vi "test Total Channel Count.vi"(8 "error in (no error)":errorcluster, 11 "TestCase in":refnum<class "Configuration Tests.lvclass">) -> (0 "error out":errorcluster, 3 "TestCase out":refnum<class "Configuration Tests.lvclass">)   [LabVIEW 2017, in "Configuration Tests.lvclass"]
uses:
  Configuration Tests.lvclass
  Mock Classes/Transfer/Mock Transfer.lvclass
  C:/github/data-sharing-framework/Data Sharing Framework Core/Engine/Classes/Transfer/Transfer.lvclass
  Configuration/Public/Controls/DSF Engine Channel Configuration.ctl
  Configuration/Public/Controls/DSF Data Type.ctl
  <vilib>/addons/_JKI Toolkits/VI Tester/TestCase.llb/TestCase.lvclass
  Engine/Classes/Transfer/Transfer.lvclass
  DSF Core.lvlib
  C:/Program Files (x86)/National Instruments/LabVIEW 2017/vi.lib/addons/_JKI Toolkits/VI Tester/TestCase.llb/TestCase.lvclass
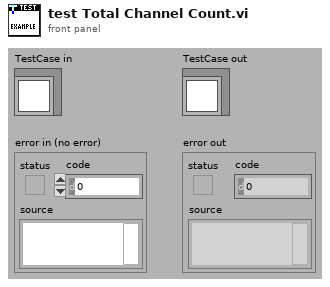
[diagram p1: front panel]
types:
  T1 = typedef "DSF Core.lvlib/DSF Engine Channel Configuration.ctl" = cluster{"engine offset":u64, "name":string, "data type":T2, "count":u64, "buffer offset":u64}
  T2 = typedef "DSF Core.lvlib/DSF Data Type.ctl" = enum8{"Bool", "SGL", "DBL", "I8", "I16", "I32", "I64", "U8", "U16", "U32", "U64"}
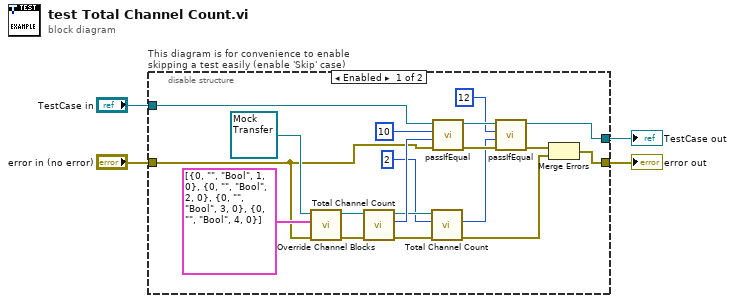
[diagram p0: block diagram]
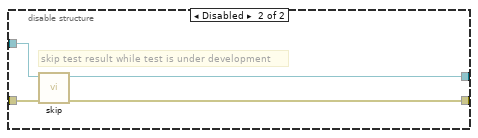
[diagram p2: hidden frame]
diagram:
  n1 = disable-structure "This diagram is for convenience to enable skipping a test easily (enable 'Skip' case)" shown="Enabled" {
    disable-tunnel: "TestCase in" -> [w18 w27]
    disable-tunnel: [w14 w25] -> w1
    disable-tunnel: [w11 w26] -> w3
    disable-tunnel: "error in (no error)" -> [w10 w24]
    frame Enabled {
      n2 = call "Override Channel Blocks.vi"("error in (no error)"=w10, "channel blocks"=T1[] [{"engine offset"=0, "name"="", "data type"=enum."Bool", "count"=1, "buffer offset"=0}, {"engine offset"=0, "name"="", "data type"=enum."Bool", "count"=2, "buffer offset"=0}, {"engine offset"=0, "name"="", "data type"=enum."Bool", "count"=3, "buffer offset"=0}, {"engine offset"=0, "name"="", "data type"=enum."Bool", "count"=4, "buffer offset"=0}], "Mock Transfer in"=refnum<class "Mock Transfer.lvclass"> refnum) -> ("error out"=w20:errorcluster, "Mock Transfer out"=w21:refnum<class "Mock Transfer.lvclass">)  [unwired: 7 in]
      n3 = call "Total Channel Count.vi"("error in (no error)"=w20, "Transfer in"=w21) -> ("error out"=w9:errorcluster, "total channel count"=w13:u64, "Transfer out"=w7:refnum<class "Mock Transfer.lvclass">)  [unwired: 7 in]
      n4 = call "Total Channel Count.vi"("error in (no error)"=w9, "previous total channel count (0)"=u64 2, "Transfer in"=w7) -> ("error out"=w8:errorcluster, "total channel count"=w5:u64)  [unwired: 6 in, 1 out]
      n5 = call-dynamic "passIfEqual.vi"("error in (no error)"=w10, "y"=w13, "x"=u64 10 ("total channel count"), "TestCase in"=w18) -> ("error out"=w19:errorcluster, "TestCase out"=w15:refnum<class "Configuration Tests.lvclass">)  [unwired: 6 in]
      n6 = call-dynamic "passIfEqual.vi"("error in (no error)"=w19, "y"=w5, "x"=u64 12 ("total channel count"), "TestCase in"=w15) -> ("error out"=w16:errorcluster, "TestCase out"=w14:refnum<class "Configuration Tests.lvclass">)  [unwired: 6 in]
      n7 = Merge Errors(w16, w8) -> (w11:errorcluster)
    }
    frame Disabled {
      # "skip test result while test is under development"
      n8 = call <vilib>:"skip.vi"("error in (no error)"=w24, "TestCase in"=w27) -> ("error out"=w26:errorcluster, "TestCase out"=w25:refnum<class "Configuration Tests.lvclass">)  [unwired: 8 in]
    }
  }
  "error out" <- w3
  "TestCase out" <- w1
